vi "Configure Multi Eval Meas PVT Enabled.vi"(8 "error in (no error)":errorcluster, 9 "Power vs Time (On)":bool=TRUE, 10 "Instance (1)":i32=1, 11 "VISA resource name":refnum<visa-resource-name>) -> (0 "error out":errorcluster, 3 "VISA resource name out":refnum<visa-resource-name>)   [LabVIEW 2020, in "Rohde&Schwarz CMP LR WPAN Measurement.lvlib"]
doc: "Enables or disables the evaluation of Power vs Time results in the multi-evaluation measurement.\n\nAttribute:\nRSCMPLRWM_ATTR_MULTIEVAL_PVT_ENABLED\n\nRemote-control command:\nCONFigure:WPAN:MEAS<i>:MEValuation:RESult:PVTime"
uses:
  <instrlib>/Rohde&Schwarz CMP LR WPAN Measurement/Rohde&Schwarz CMP LR WPAN Measurement.lvlib
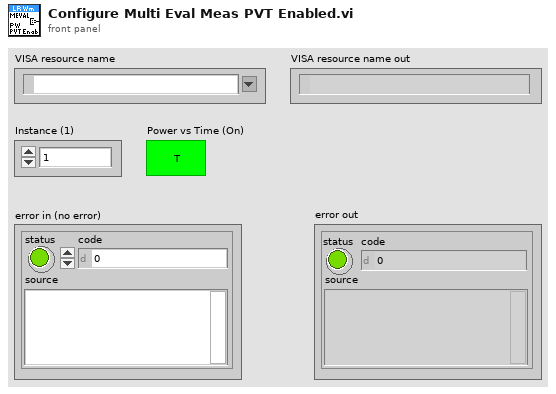
[diagram p1: front panel]
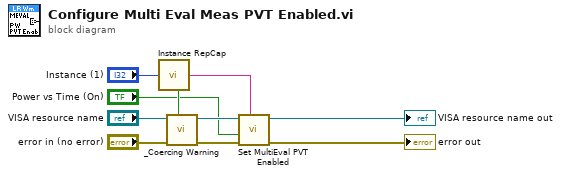
[diagram p0: block diagram]
diagram:
  n1 = call <instrlib>:"Instance RepCap.vi"("Instance In"="Instance (1)") -> ("In Range?"=w9:bool, "RepCap Identifier Out"=w10:string)  [unwired: 1 in]
  n2 = call <instrlib>:"_Coercing Warning.vi"("In Range?"=w9, "error in (no error)"="error in (no error)", "VISA resource name"="VISA resource name") -> ("error out"=w6:errorcluster, "VISA resource name out"=w5:refnum<visa-resource-name>)  [unwired: 7 in]
  n3 = call "Set MultiEval PVT Enabled"("Repeated Capabilities"=w10, "error in (no error)"=w6, "MultiEval PVT Enabled (OFF)"="Power vs Time (On)", "instrument handle"=w5) -> ("error out"=→"error out":errorcluster, "instrument handle out"=→"VISA resource name out":refnum<visa-resource-name>)  [unwired: 6 in]
